vi "SSC DCPower Configure Source Mode.vi"(0 "DCPower SSC in":T2[](array[typedef]), 5 "Source Mode":T1=1020 items=["Single Point"=1020, "Sequence"=1021], 11 "error in":errorcluster) -> (4 "DCPower SSC out":T2[](array[typedef]), 15 "error out":errorcluster)   [LabVIEW 2019]
doc: "This VI configures the sourcing mode of the instrument sessions. The tasks must be aborted when calling this method."
uses:
  SSC DCPower.ctl
  <instrlib>/niDCPower/nidcpower.llb/niDCPower Source Mode.ctl
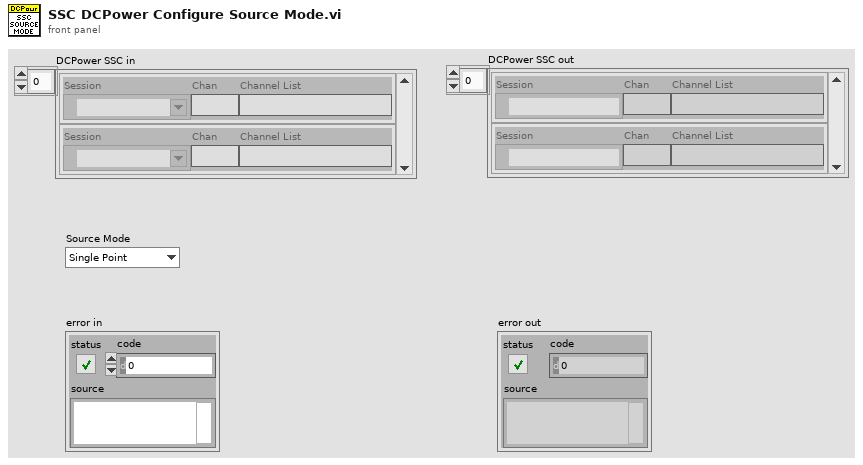
[diagram p1: front panel]
types:
  T1 = typedef "niDCPower Source Mode.ctl" = i32
  T2 = typedef "SSC DCPower.ctl" = cluster{"Session":refnum<k15>, "Chan":string, "Channel List":string}
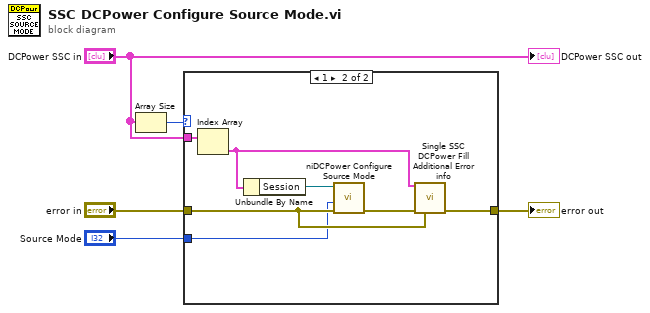
[diagram p0: block diagram]
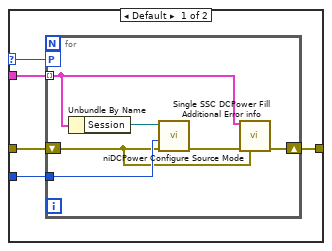
[diagram p2: hidden frame]
diagram:
  n1 = Array Size(array="DCPower SSC in") -> (size(s)=w3:i32)
  n2 = case shown="1" w3 {
    selector: w3 -> [w8 _]
    tunnel: [w10 w23] -> w5
    tunnel: "error in" -> [w9 w22]
    tunnel: "DCPower SSC in" -> [w7 w21]
    tunnel: "Source Mode" -> [w6 w20]
    frame Default {
      n3 = for {
        workers-P: w8 -> [_]
        tunnel: w7 -> [w12] mode=indexing
        shift-right: [w13] -> w10
        shift-left: w9 -> [w11]
        tunnel: w6 -> [w14]
        n4 = Unbundle By Name(w12) -> ("Session"=w16:refnum<k15>)
        n5 = call <instrlib>:"niDCPower Configure Source Mode.vi"("error in (no error)"=w11, "source mode"=w14, "instrument handle"=w16) -> ("error out"=w15:errorcluster)  [unwired: 7 in, 1 out]
        n6 = call "Single SSC DCPower Fill Additional Error info.vi"("DCPower SSC in"=w12, "error in"=w15, "previous error in"=w11) -> ("error out"=w13:errorcluster)  [unwired: 12 in]
      }
    }
    frame 1 {
      n7 = Index Array(array=w21) -> (element=w17:T2)  [unwired: 1 in]
      n8 = Unbundle By Name(w17) -> ("Session"=w19:refnum<k15>)
      n9 = call <instrlib>:"niDCPower Configure Source Mode.vi"("error in (no error)"=w22, "source mode"=w20, "instrument handle"=w19) -> ("error out"=w18:errorcluster)  [unwired: 7 in, 1 out]
      n10 = call "Single SSC DCPower Fill Additional Error info.vi"("DCPower SSC in"=w17, "error in"=w18, "previous error in"=w22) -> ("error out"=w23:errorcluster)  [unwired: 12 in]
    }
  }
  "error out" <- w5
  "DCPower SSC out" <- "DCPower SSC in"
